vi "Escape String.vi"(10 "Message In":string) -> (2 "Message Out":string)   [LabVIEW 2011, in "StatD Interface.lvclass"]
uses:
  StatD Interface.lvclass
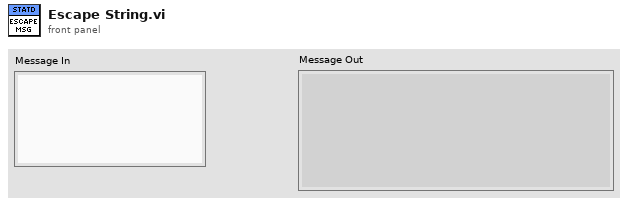
[diagram p1: front panel]
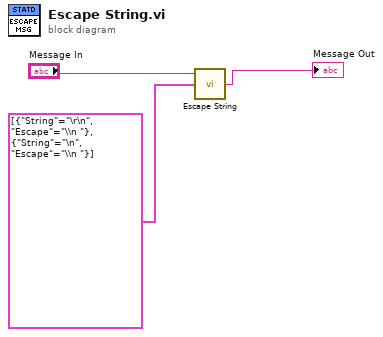
[diagram p0: block diagram]
diagram:
  n1 = call <vilib>:"Escape String.vi"("Escapes"=cluster{"String":string, "Escape":string}[] [{"String"="\r\n", "Escape"="\\n "}, {"String"="\n", "Escape"="\\n "}], "String in"="Message In") -> ("String out"=→"Message Out":string)  [unwired: 1 in]
